vi "Global_SM Write_Data Out.vi"() -> ()   [LabVIEW 2017]
uses:
  TypeDef/ENUM_Drive_ACT Loop_Mode.ctl
  TypeDef/ENUM_Drive_Profile_CMD.ctl
  TypeDef/CLUSTER_Left and Right.ctl
panel:
  out "WC_Drive_SM_Zero_Encoders":bool
  out "WC_Drive_SM_Encoder_target_position":dbl
  in  "WC_Drive_SM_VBus":T1
  in  "WC_Drive_SM_ProfileCmd":T2
  in  "WC_Drive_SM_Mode":T3
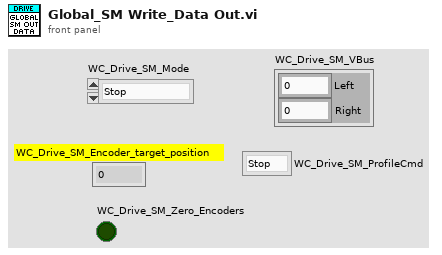
[diagram p1: front panel]
types:
  T1 = typedef "CLUSTER_Left and Right.ctl" = cluster{"Left":dbl, "Right":dbl}
  T2 = typedef "ENUM_Drive_Profile_CMD.ctl" = enum16{"Stop", "Setup", "Run"}
  T3 = typedef "ENUM_Drive_ACT Loop_Mode.ctl" = enum16{"Stop", "Position", "VBus", "Profile"}
diagram:
